vi "SendUpstreamMsg.vi"(8 "error in (no error)":errorcluster, 10 "UpstreamMsg":refnum<class "UpstreamMsgParent.lvclass">, 11 "ServiceManager-Comms in":refnum<class "ServiceManager-Comms.lvclass">) -> (0 "error out":errorcluster, 3 "ServiceManager-Comms out":refnum<class "ServiceManager-Comms.lvclass">)   [LabVIEW 2020, in "ServiceManager.lvlib" / "ServiceManager-Comms.lvclass"]
uses:
  ServiceManager-Comms.lvclass
  ServiceManager/UpstreamMsg/UpstreamMsgParent/UpstreamMsgParent.lvclass
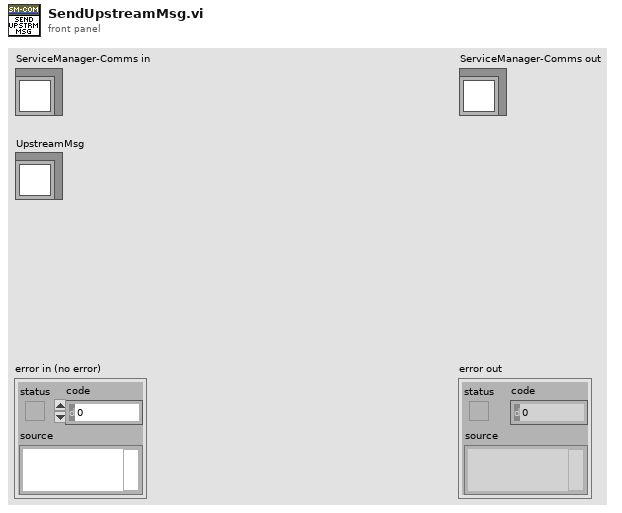
[diagram p1: front panel]
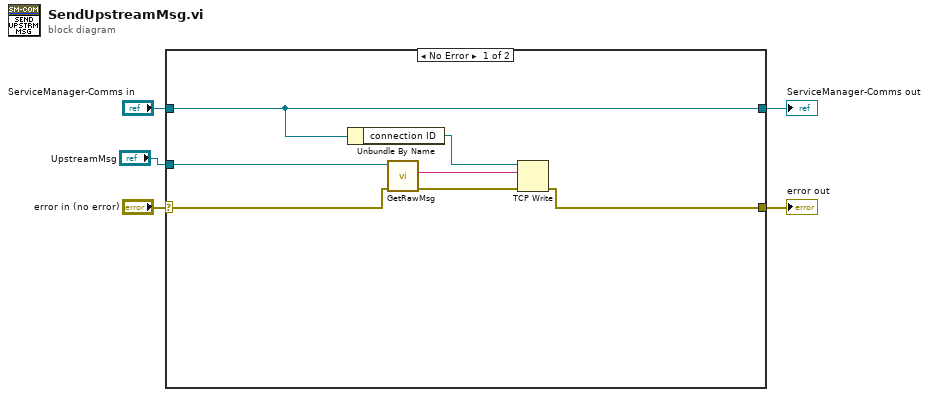
[diagram p0: block diagram]
diagram:
  n1 = case shown="No Error" "error in (no error)" {
    selector: "error in (no error)" -> [w11 w14]
    tunnel: [w7 w14] -> w4
    tunnel: [w6 w13] -> w2
    tunnel: "ServiceManager-Comms in" -> [w6 w13]
    tunnel: "UpstreamMsg" -> [w12 _]
    frame No Error {
      n2 = Unbundle By Name(w6) -> ("connection ID"=w10:refnum<k5>)
      n3 = call-dynamic "GetRawMsg.vi"("error in (no error)"=w11, "UpstreamMsgParent in"=w12) -> ("error out"=w9:errorcluster, "Msg"=w8:string)  [unwired: 7 in, 1 out]
      n4 = TCP Write(connection ID=w10, data in=w8, error in (no error)=w9) -> (error out=w7:errorcluster)  [unwired: 1 in, 2 out]
    }
    frame Error {
    }
  }
  "error out" <- w4
  "ServiceManager-Comms out" <- w2
